vi "Send Configure Width Trigger Source [WT].vi"(2 "width high threshold (2.0 E-9 V)":dbl[unit]=2e-09 format="%^.3e", 4 "width low threshold (1.0 E-9 V)":dbl[unit]=1e-09 format="%^.3e", 5 "width polarity (Positive)":i32(ring)=1 items=["Positive"=1, "Negative"=2], 6 "width condition (Within)":i32(ring)=1 items=["Within"=1, "Outside"=2], 7 "Message Priority (Normal)":T1=enum."Normal", 8 "error in (no error)":errorcluster, 9 "trigger level (0.0 V)":dbl[unit] format="%.3f", 10 "trigger source (\"CHANNEL1\")":string(combo)="CHANNEL1", 11 "Message Enqueuer":refnum<class "Message Enqueuer.lvclass">) -> (0 "error out":errorcluster, 3 "Message Enqueuer out":refnum<class "Message Enqueuer.lvclass">)   [LabVIEW 2015, in "CS++Scope.lvlib" / "Configure Width Trigger Source [WT] Msg.lvclass"]
doc: "Sends the <B>CS++Scope.lvlib:Configure Width Trigger Source [WT] Msg.lvclass</B> message.\n\n<B>CS++Scope.lvlib:CS++Scope.lvclass:Configure Width Trigger Source [WT].vi</B> Description:\n\nThis VI configures the width trigger. A width trigger occurs when the oscilloscope detects a positive or negative pulse with a width between, or optionally outside, the width thresholds. You specify the width thresholds with the Width Low Threshold and Width High Threshold parameters. You specify whether the oscilloscope triggers on pulse widths that are within or outside the width thresholds with the Width Condition parameter. You specify the polarity of the pulse with the Width Polarity parameter. The trigger does not actually occur until the edge of a pulse that corresponds to the Width Low Threshold, Width High Threshold, Width Condition, and Width Polarity crosses the threshold you specify in the Trigger Level parameter.\n\nNote (1) This VI affects instrument behavior only if the trigger type is IVISCOPE_VAL_WIDTH_TRIGGER. Call the IviScope Configure Trigger and IviScope Configure Trigger Coupling VIs to set the trigger type and trigger coupling before calling this VI.\n(2) This VI is part of the IviScopeWidthTrigger [WT] extension group."
uses:
  Configure Width Trigger Source [WT] Msg.lvclass
  <vilib>/ActorFramework/Message Enqueuer/Message Enqueuer.lvclass
  <vilib>/ActorFramework/Message Enqueuer/Message Priority.ctl
  Configure Width Trigger Source [WT] Msg.lvclass/Configure Width Trigger Source [WT] Msg.ctl
  <vilib>/ActorFramework/Message Enqueuer/Message Enqueuer.lvclass/Message Enqueuer.ctl
  <vilib>/ActorFramework/Message Priority Queue/Priority Enqueue.vi
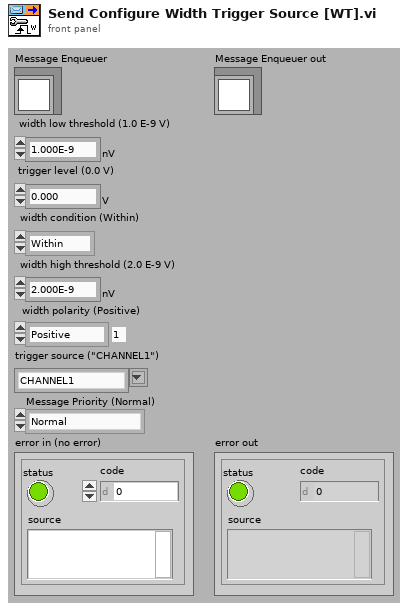
[diagram p1: front panel]
types:
  T1 = typedef "Actor Framework.lvlib/Message Enqueuer.lvclass/Message Priority.ctl" = enum16{"Low", "Normal", "High"}
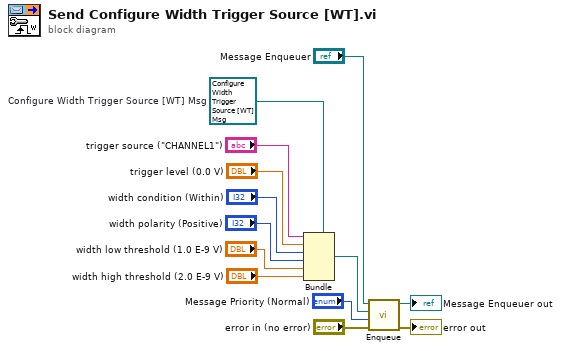
[diagram p0: block diagram]
diagram:
  w7 = refnum<class "Configure Width Trigger Source [WT] Msg.lvclass"> refnum  # Configure Width Trigger Source [WT] Msg
  n1 = Bundle(cluster=w7, "trigger source (\"CHANNEL1\")", "trigger level (0.0 V)", "width condition (Within)", "width polarity (Positive)", "width low threshold (1.0 E-9 V)", "width high threshold (2.0 E-9 V)") -> (w10:refnum<class "Configure Width Trigger Source [WT] Msg.lvclass">)
  n2 = call <vilib>:"Enqueue.vi"("error in (no error)"="error in (no error)", "Message Priority (Normal)"="Message Priority (Normal)", "Message"=w10, "Message Enqueuer in"="Message Enqueuer") -> ("error out"=→"error out":errorcluster, "Message Enqueuer out"=→"Message Enqueuer out":refnum<class "Message Enqueuer.lvclass">)  [unwired: 6 in]
